vi "TWM Client Cmd Define Multiplexer Sequence.vi"(5 "timeout [ms]":i32=5000, 7 "end of packet key":string="TWM:command:EndOfPacket", 8 "error in":errorcluster, 10 "sequence item strings":string[](array[string]), 11 "handle":i32) -> (0 "error out":errorcluster, 3 "handle out":i32)   [LabVIEW 2020, in "TWM Client.lvlib"]
doc: "This will define multiplexer sequence. It's equivalent to manual setup in multiplexer panel. Sequence tag names must exist for currently selected multiplexer!"
uses:
  TWM Client.lvlib
  1D String.vi
  infolib.lvlib
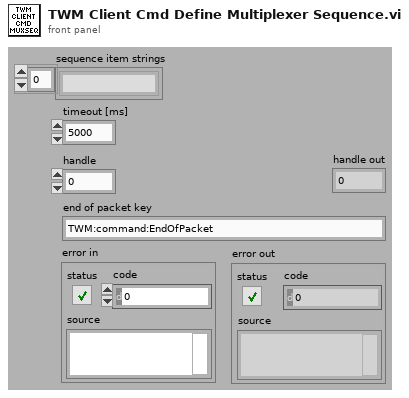
[diagram p1: front panel]
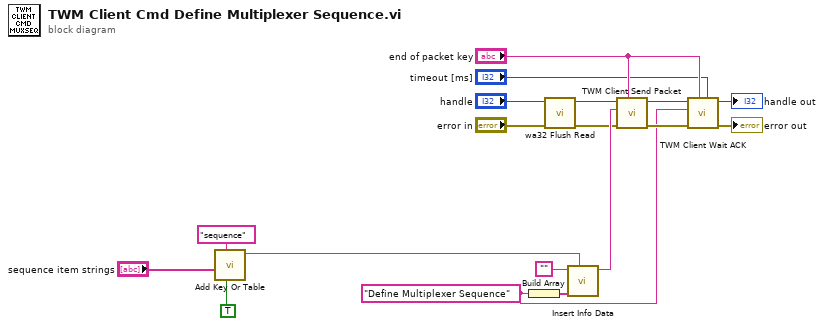
[diagram p0: block diagram]
diagram:
  w11 = "Define Multiplexer Sequence" ("section name")
  n1 = call-poly "Add Key Or Table.vi"("collumn vector (F)"=TRUE, "key description"="sequence", "string"="sequence item strings") -> ("info data out"=w5:string)  [unwired: 7 in, 1 out]
  n2 = Build Array(w11) -> (w17:string[])
  n3 = call "wa32 Flush Read.vi"("error in"="error in", "handle"="handle") -> ("error out"=w3:errorcluster, "handle out"=w2:i32)  [unwired: 7 in, 1 out]
  n4 = call "Insert Info Data.vi"("info data to insert"=w5, "sections"=w17, "info data"="") -> ("info data out"=w18:string)  [unwired: 7 in, 1 out]
  n5 = call "TWM Client Send Packet.vi"("end of packet key"="end of packet key", "error in"=w3, "command string"=w18, "handle"=w2) -> ("error out"=w13:errorcluster, "handle out"=w10:i32)  [unwired: 6 in]
  n6 = call "TWM Client Wait ACK.vi"("timeout [ms] (3000)"="timeout [ms]", "key string"="end of packet key", "error in"=w13, "command header"=w11, "handle"=w10) -> ("error out"=→"error out":errorcluster, "handle out"=→"handle out":i32)  [unwired: 5 in]
